vi "ADCCalc.vi"(1 "Rsense":dbl, 2 "Gain":dbl, 3 "DATA":u16) -> (0 "NumOut":dbl)   [LabVIEW 2010]
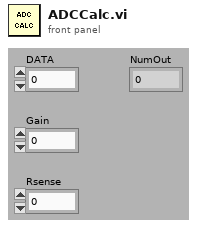
[diagram p1: front panel]
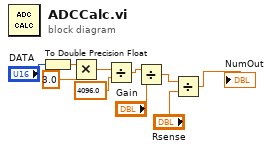
[diagram p0: block diagram]
diagram:
  n1 = To Double Precision Float(number="DATA") -> (double precision float=w2:dbl)
  n2 = Multiply(x=w2, y=3.0) -> (x*y=w4:dbl)
  n3 = Divide(x=w4, y=4096.0) -> (x/y=w6:dbl)
  n4 = Divide(x=w6, y="Gain") -> (x/y=w8:dbl)
  n5 = Divide(x=w8, y="Rsense") -> (x/y=→"NumOut":dbl)
